vi "Connect to PS3 Controller.vi"(10 "device ID":i32) -> (0 "error out":errorcluster, 2 "device ID 2":refnum<k1>, 3 "element":T1)   [LabVIEW 2014]
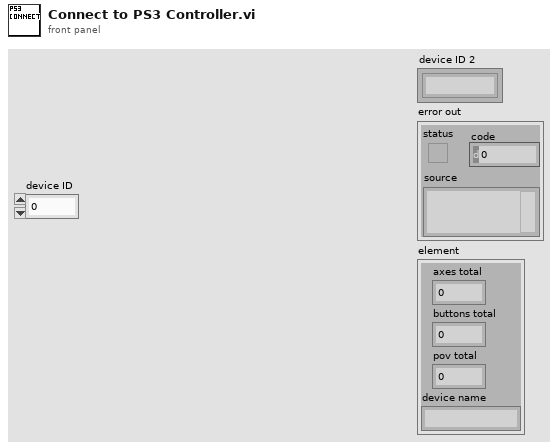
[diagram p1: front panel]
types:
  T1 = cluster{"axes total":u32, "buttons total":u32, "pov total":u32, "device name":string}
  T2 = cluster{"axes total":u32, "buttons total":u32, "pov total":u32, "device name":string}[]
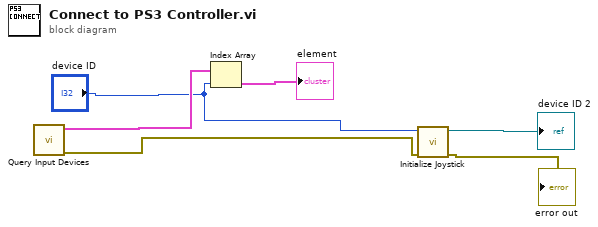
[diagram p0: block diagram]
diagram:
  n1 = call <vilib>:"Query Input Devices.vi"() -> ("error out"=w4:errorcluster, "joystick info"=w6:T2)  [unwired: 8 in, 2 out]
  n2 = Index Array(array=w6, index="device ID") -> (element=→"element":T1)
  n3 = call <vilib>:"Initialize Joystick.vi"("error in (no error)"=w4, "device index"="device ID") -> ("error out"=→"error out":errorcluster, "device ID"=→"device ID 2":refnum<k1>)  [unwired: 8 in]
